vi "entryParaChk.vi"(7 "indexSec":string, 8 "error in":errorcluster, 9 "Row number":u32, 10 "Tbl Refnum in":refnum<vi>, 11 "Tree Refnum in":refnum<vi>) -> (0 "error out":errorcluster, 1 "Check result":string="√", 2 "Tbl Refnum out":refnum<vi>, 3 "Tree Refnum out":refnum<vi>)   [LabVIEW 2010]
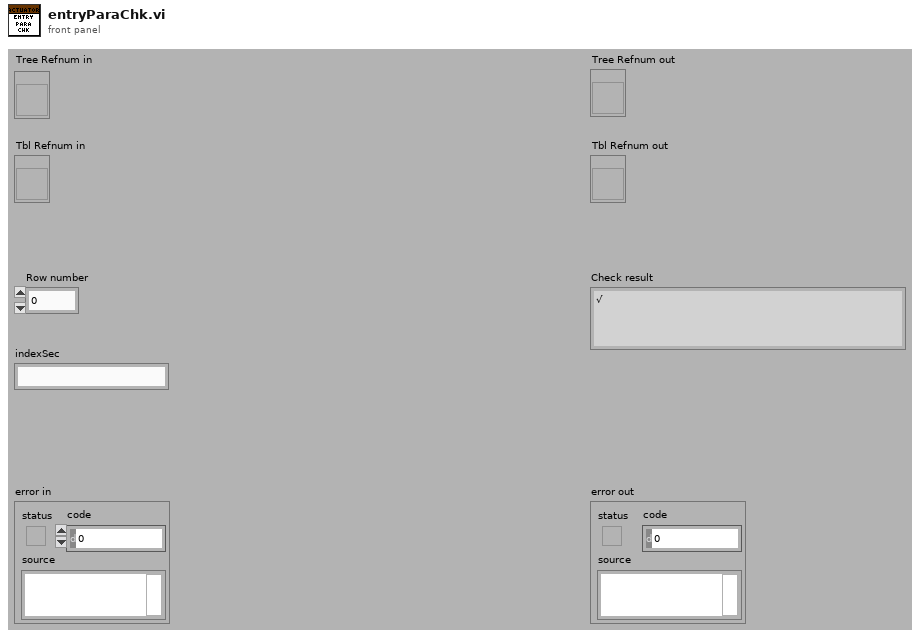
[diagram p1: front panel]
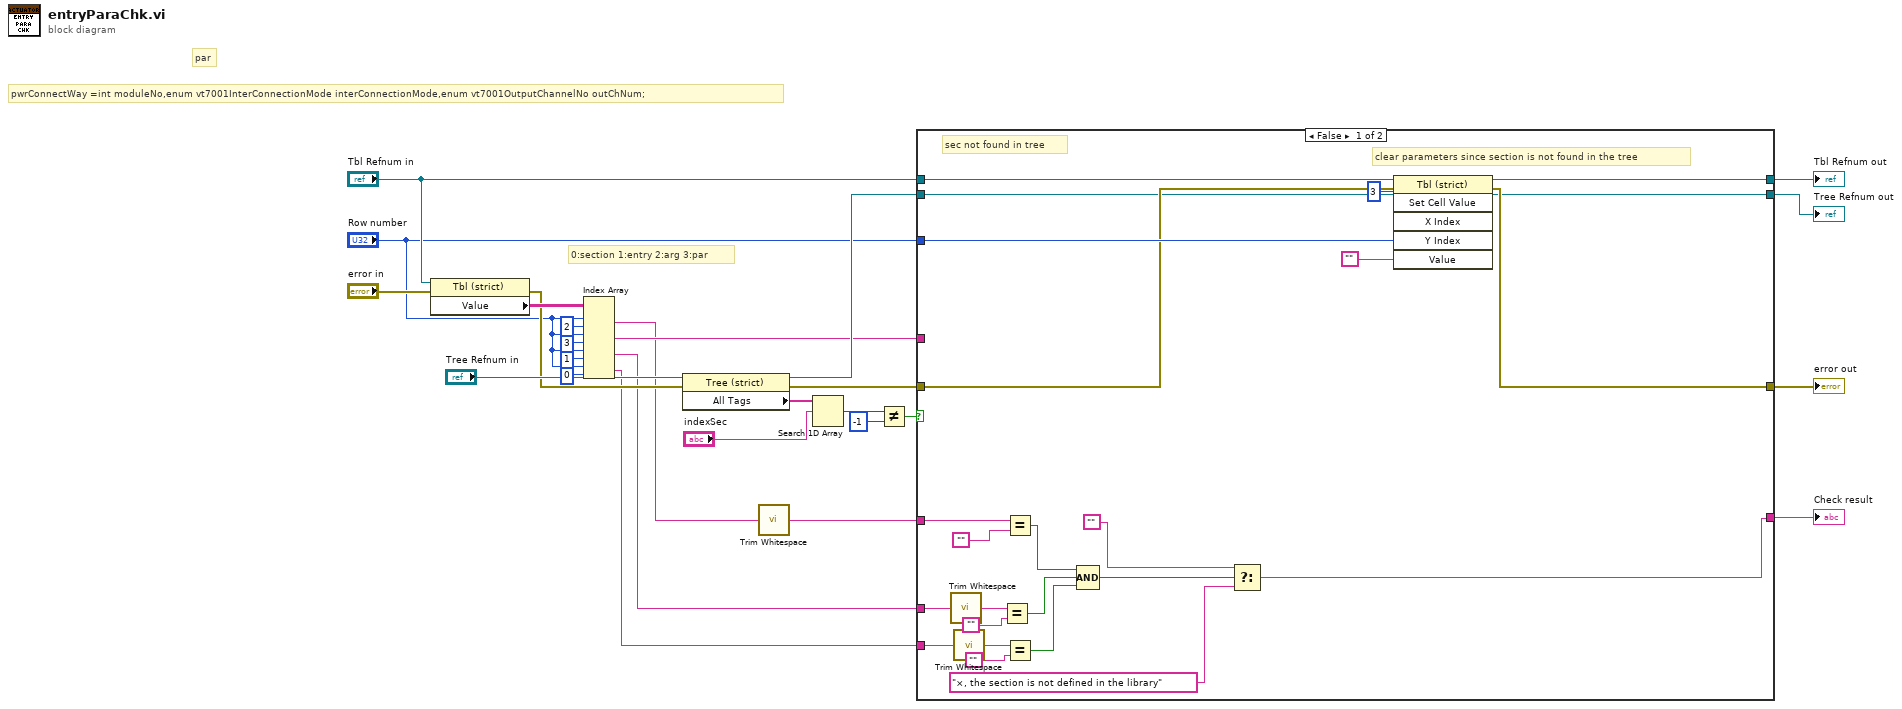
[diagram p0: block diagram]
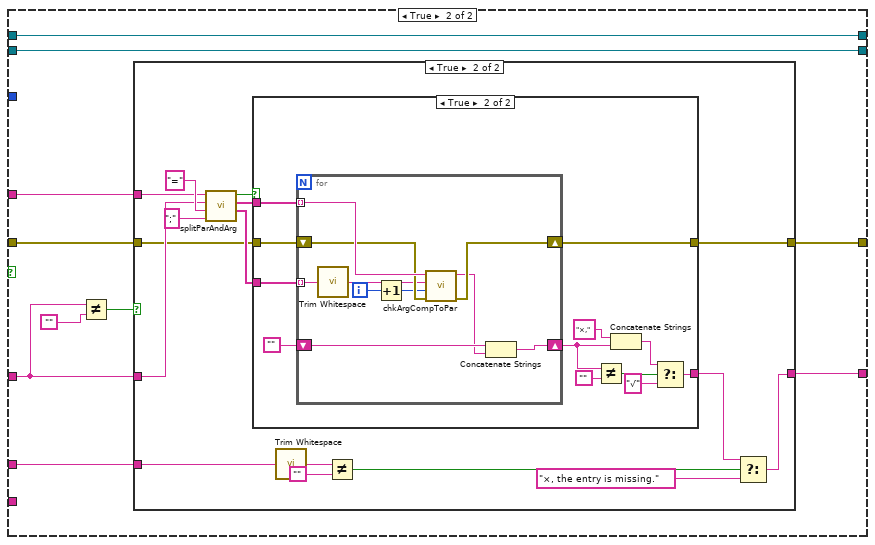
[diagram p2: hidden frame]
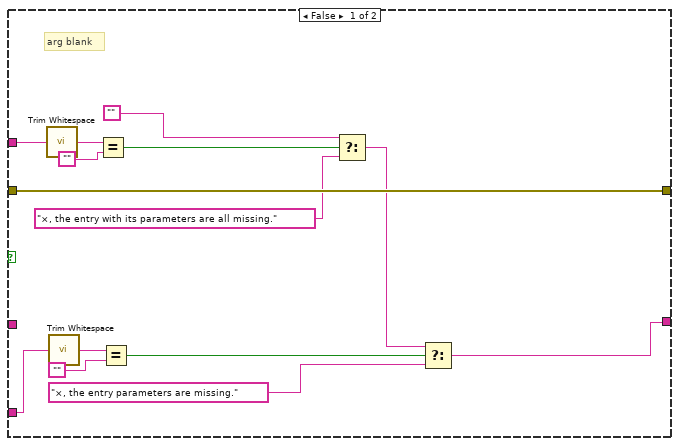
[diagram p3: hidden frame]
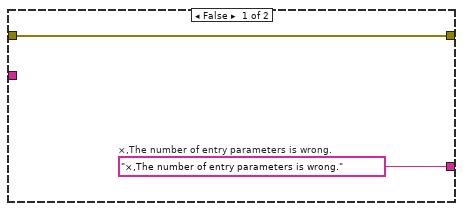
[diagram p4: hidden frame]
diagram:
  # "pwrConnectWay =int moduleNo,enum vt7001InterConnectionMode interConnectionMode,enum vt7001OutputChannelNo outChNum;"
  # "par"
  # "0:section 1:entry 2:arg 3:par"
  n1 = property class="Tbl (strict)"(reference="Tbl Refnum in", error in="error in") -> (error out=w12:errorcluster, "Value"=w15:string[][])  [unwired: 1 out]
  n2 = Index Array(array=w15, index (row) #1="Row number", index (col) #1=2 ("index (col)"), index (row) #2="Row number", index (col) #2=3 ("disabled index (col)"), index (row) #3="Row number", index (col) #3=1 ("disabled index (col)"), index (row) #4="Row number", index (col) #4=0 ("disabled index (col)")) -> (element #1=w7:string, element #2=w8:string, element #3=w4:string, element #4=w1:string)
  n3 = property on="Property Node" class="Tree (strict)"(reference="Tree Refnum in", error in=w12) -> (reference out=w18:refnum<vi>, error out=w19:errorcluster, "All Tags"=w22:string[])
  n4 = call <vilib>:"Trim Whitespace.vi"("string"=w7) -> ("trimmed string"=w11:string)  [unwired: 1 in]
  n5 = Search 1D Array(1D array=w22, element="indexSec") -> (index of element=w21:i32)  [unwired: 1 in]
  n6 = Not Equal?(x=w21, y=-1) -> (x != y?=w26:bool)
  n7 = case shown="False" w26 {
    tunnel: w8 -> [_ w59]
    tunnel: w11 -> [w34 w50]
    tunnel: w19 -> [w43 w58]
    tunnel: [w27 w57] -> w25
    tunnel: [w46 w56] -> w24
    tunnel: "Tbl Refnum in" -> [w44 w52]
    tunnel: "Row number" -> [w45 _]
    tunnel: [w47 w52] -> w23
    tunnel: w18 -> [w42 w53]
    tunnel: [w42 w53] -> w17
    tunnel: w4 -> [w40 w51]
    tunnel: w1 -> [w35 _]
    frame False {
      # "clear parameters since section is not found in the tree"
      # "sec not found in tree"
      n8 = call <vilib>:"Trim Whitespace.vi"("string"=w40) -> ("trimmed string"=w36:string)  [unwired: 1 in]
      n9 = call <vilib>:"Trim Whitespace.vi"("string"=w35) -> ("trimmed string"=w37:string)  [unwired: 1 in]
      n10 = Equal?(x=w36, y="") -> (x = y?=w32:bool)
      n11 = Equal?(x=w34, y="") -> (x = y?=w33:bool)
      n12 = Equal?(x=w37, y="") -> (x = y?=w31:bool)
      n13 = Compound Arithmetic op=AND(w33, w32, w31) -> (w30:bool)
      n14 = Select(t="", s=w30, f="×, the section is not defined in the library") -> (s? t:f=w27:string)
      n15 = invoke class="Tbl (strict)" method="Set Cell Value"(reference=w44, error in=w43, "X Index"=u32 3, "Y Index"=w45, "Value"="") -> (reference out=w47:refnum<vi>, error out=w46:errorcluster)  [unwired: 1 in, 4 out]
    }
    frame True {
      n16 = Not Equal?(x=w50, y="") -> (x != y?=w54:bool)
      n17 = case shown="True" w54 {
        tunnel: w59 -> [w66 w75]
        tunnel: w50 -> [_ w86]
        tunnel: w58 -> [w73 w82]
        tunnel: [w69 w76] -> w57
        tunnel: [w73 w89] -> w56
        tunnel: w51 -> [w68 w74]
        frame False {
          # "arg blank"
          n18 = call <vilib>:"Trim Whitespace.vi"("string"=w66) -> ("trimmed string"=w65:string)  [unwired: 1 in]
          n19 = call <vilib>:"Trim Whitespace.vi"("string"=w68) -> ("trimmed string"=w72:string)  [unwired: 1 in]
          n20 = Equal?(x=w65, y="") -> (x = y?=w63:bool)
          n21 = Equal?(x=w72, y="") -> (x = y?=w70:bool)
          n22 = Select(t="", s=w63, f="×, the entry with its parameters are all missing.") -> (s? t:f=w60:string)
          n23 = Select(t=w60, s=w70, f="×, the entry parameters are missing.") -> (s? t:f=w69:string)
        }
        frame True {
          n24 = call "splitParAndArg.vi"("paraEndMark"=";" ("regular expression"), "paraStartMark"="=" ("regular expression"), "allArguments"=w86, "allParameters"=w75) -> ("argArray"=w84:string[], "paraArray"=w85:string[], "sameNum?"=w83:bool)  [unwired: 5 in]
          n25 = case shown="True" w83 {
            tunnel: w85 -> [_ w103]
            tunnel: w84 -> [_ w102]
            tunnel: [w91 w97] -> w78
            tunnel: w82 -> [w90 w96]
            tunnel: [w90 w95] -> w89
            frame False {
              w91 = "×,The number of entry parameters is wrong."  # ×,The number of entry parameters is wrong.
            }
            frame True {
              n26 = for {
                tunnel: w103 -> [w113] mode=indexing
                tunnel: w102 -> [w107] mode=indexing
                shift-right: [w111] -> w93
                shift-left: "" -> [w112]
                shift-right: [w109] -> w95
                shift-left: w96 -> [w110]
                i -> [w108]
                n27 = call <vilib>:"Trim Whitespace.vi"("string"=w107) -> ("trimmed string"=w106:string)  [unwired: 1 in]
                n28 = Increment(x=w108) -> (x+1=w105:i32)
                n29 = call "chkArgCompToPar.vi"("error in"=w110, "argSN"=w105, "arg"=w106, "par"=w113) -> ("error out"=w109:errorcluster, "judgement"=w104:string)  [unwired: 6 in]
                n30 = Concatenate Strings(w112, w104) -> (w111:string)
              }
              n31 = Not Equal?(x=w93, y="") -> (x != y?=w99:bool)
              n32 = Concatenate Strings("×,", w93) -> (w92:string)
              n33 = Select(t=w92, s=w99, f="√") -> (s? t:f=w97:string)
            }
          }
          n34 = call <vilib>:"Trim Whitespace.vi"("string"=w74) -> ("trimmed string"=w81:string)  [unwired: 1 in]
          n35 = Not Equal?(x=w81, y="") -> (x != y?=w79:bool)
          n36 = Select(t=w78, s=w79, f="×, the entry is missing.") -> (s? t:f=w76:string)
        }
      }
    }
  }
  "Check result" <- w25
  "error out" <- w24
  "Tbl Refnum out" <- w23
  "Tree Refnum out" <- w17
